vi "TSM Get Ref Mic Settings.vi"(0 "TSM context":T1, 11 "error in (no error)":errorcluster) -> (3 "current excitation (4mA)":dbl=0.004 format="%#_13g", 4 "TSM context Out":T1, 6 "Sampling Rate (Hz)":dbl format="%#_13g", 8 "Samples per channel":i32=1000, 10 "max dB SPL":dbl=132.0 format="%#_13g", 15 "error out":errorcluster)   [LabVIEW 2020]
doc: "Get the settings from Spec sheet using TSM context"
uses:
  <vilib>/NI_TestStand_SemiconductorModule/NI_TestStand_Semiconductor_Module.lvlibp/PinMap/General/SemiconductorModuleContext.ctl
  <vilib>/NI_TestStand_SemiconductorModule/NI_TestStand_Semiconductor_Module.lvlibp/PinMap/Specs/NamespacedSymbolsToValues.vi
  <vilib>/NI_TestStand_SemiconductorModule/NI_TestStand_Semiconductor_Module.lvlibp
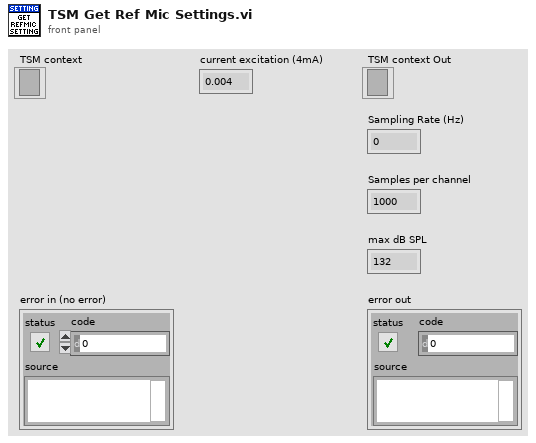
[diagram p1: front panel]
types:
  T1 = typedef "NI_TestStand_Semiconductor_Module.lvlibp/SemiconductorModuleContext.ctl" = refnum<k7>
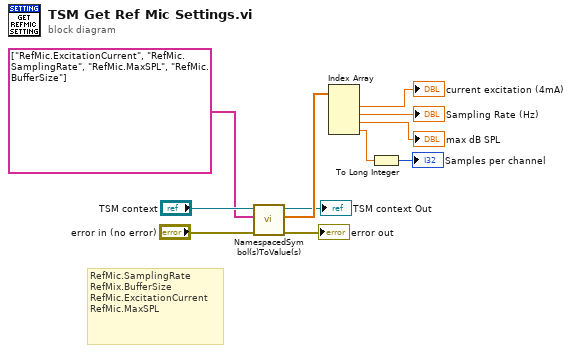
[diagram p0: block diagram]
diagram:
  # "RefMic.SamplingRate\nRefMix.BufferSize\nRefMic.ExcitationCurrent\nRefMic.MaxSPL"
  n1 = call-poly <vilib>:"NamespacedSymbol(s)ToValue(s).vi"("error in (no error)"="error in (no error)", "Symbols"=tag[] ["RefMic.ExcitationCurrent", "RefMic.SamplingRate", "RefMic.MaxSPL", "RefMic.BufferSize"], "Semiconductor Module Context"="TSM context") -> ("error out"=→"error out":errorcluster, "Values"=w8:dbl[], "Semiconductor Module Context Out"=→"TSM context Out":T1)  [unwired: 6 in]
  n2 = Index Array(array=w8) -> (element #1=→"current excitation (4mA)":dbl, element #2=→"Sampling Rate (Hz)":dbl, element #3=→"max dB SPL":dbl, element #4=w4:dbl)  [unwired: 4 in]
  n3 = To Long Integer(number=w4) -> (32bit integer=→"Samples per channel":i32)
